vi "ALG 1.vi"() -> ()   [LabVIEW 2020]
panel:
  in  "ORDEN":i32
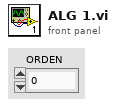
[diagram p1: front panel]
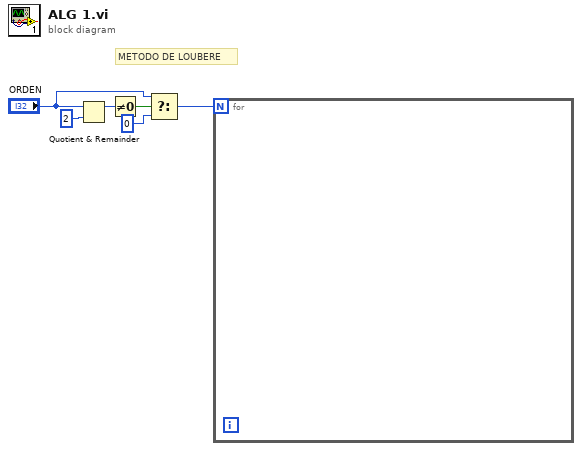
[diagram p0: block diagram]
diagram:
  # "METODO DE LOUBERE"
  n1 = Quotient & Remainder(x="ORDEN", y=2) -> (x-y*floor(x/y)=w5:i32)  [unwired: 1 out]
  n2 = Not Equal To 0?(x=w5) -> (x != 0?=w4:bool)
  n3 = Select(t="ORDEN", s=w4, f=0) -> (s? t:f=w1:i32)
  n4 = for {
    N: w1 -> [_]
  }
